vi "Class Map to Plant UML String.vi"(7 "Disabled Set":set{string}(c389), 8 "Usage":bool, 9 "Composition":bool, 10 "Inheritance":bool, 11 "Class Map":T1(c390)) -> (3 "Plant UML String":string)   [LabVIEW 2019]
uses:
  c1262000-356c-4740-a151-1e3da8a0ac02.vi
  72cd38b6-9a28-47ee-a1ef-5582ba5405b3.vi
  38964770-3a7b-4feb-bb65-44f835b9f33f.vi
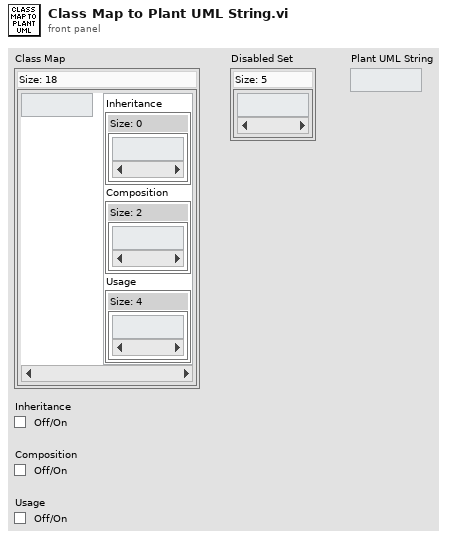
[diagram p1: front panel]
types:
  T1 = map{string, cluster{"Inheritance":set{string}, "Composition":set{string}, "Usage":set{string}}}
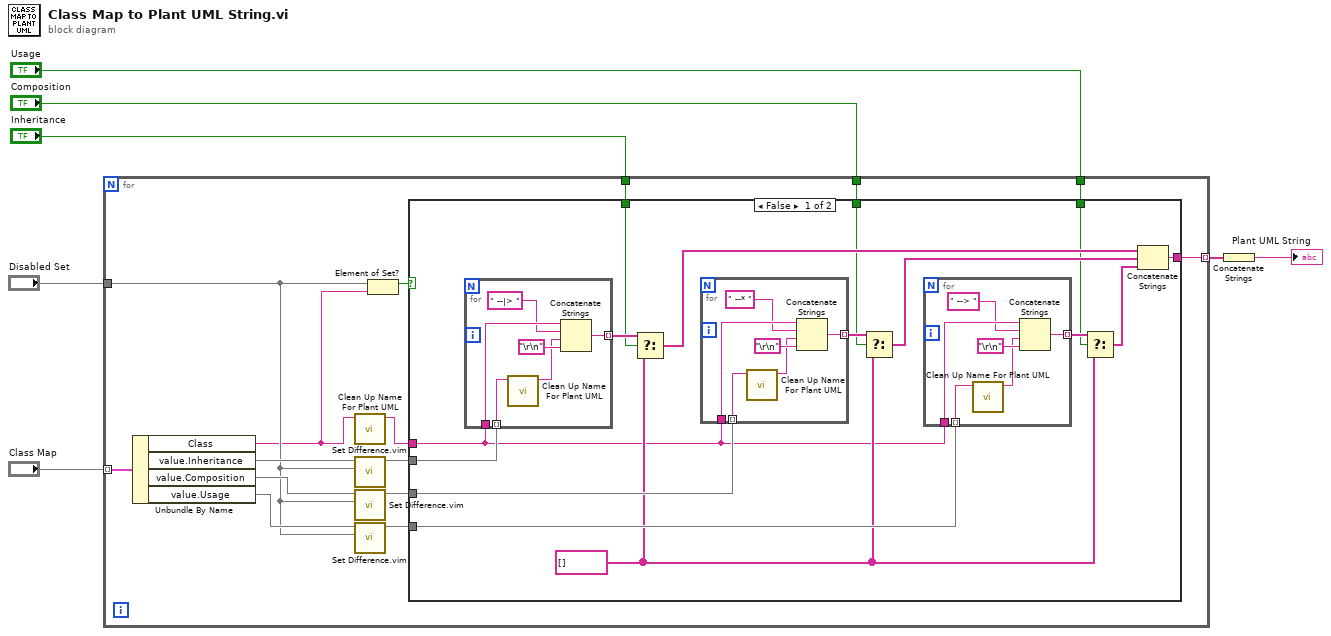
[diagram p0: block diagram]
diagram:
  n1 = for {
    tunnel: "Class Map" -> [w22] mode=indexing
    tunnel: [w21] -> w2 mode=indexing
    tunnel: "Inheritance" -> [w20]
    tunnel: "Composition" -> [w19]
    tunnel: "Usage" -> [w18]
    tunnel: "Disabled Set" -> [w10]
    n2 = Unbundle By Name(w22) -> ("Class"=w9:string, "value.Inheritance"=w16:set{string}, "value.Composition"=w13:set{string}, "value.Usage"=w11:set{string})
    n3 = call "Clean Up Name For Plant UML.vi"("Class Name"=w9) -> ("Plant UML Class Name"=w8:string)  [unwired: 10 in]
    n4 = call "Set Difference.vim"("set 2"=w10, "set 1"=w16) -> ("difference"=w15:set{string})  [unwired: 9 in]
    n5 = call "Set Difference.vim"("set 2"=w10, "set 1"=w13) -> ("difference"=w14:set{string})  [unwired: 9 in]
    n6 = call "Set Difference.vim"("set 2"=w10, "set 1"=w11) -> ("difference"=w12:set{string})  [unwired: 9 in]
    n7 = Element of Set?(10:w9, 11:w10) -> (3:w17:bool)
    n8 = case shown="False" w17 {
      tunnel: w15 -> [w37 _]
      tunnel: w14 -> [w36 _]
      tunnel: w12 -> [w35 _]
      tunnel: [w34 _] -> w21
      tunnel: w20 -> [w26 _]
      tunnel: w19 -> [w25 _]
      tunnel: w18 -> [w24 _]
      tunnel: w8 -> [w23 _]
      frame False {
        w28 = string[] [] ("f")
        n9 = for {
          tunnel: w23 -> [w55]
          tunnel: w37 -> [w51] mode=indexing
          tunnel: [w52] -> w33 mode=indexing
          n10 = call "Clean Up Name For Plant UML.vi"("Class Name"=w51) -> ("Plant UML Class Name"=w50:string)  [unwired: 10 in]
          n11 = Concatenate Strings(w55, " --|> " ("string"), w50, "\r\n") -> (w52:string)
        }
        n12 = Select(t=w33, s=w26, f=w28) -> (s? t:f=w32:string[])
        n13 = for {
          tunnel: w23 -> [w49]
          tunnel: w36 -> [w45] mode=indexing
          tunnel: [w46] -> w31 mode=indexing
          n14 = call "Clean Up Name For Plant UML.vi"("Class Name"=w45) -> ("Plant UML Class Name"=w44:string)  [unwired: 10 in]
          n15 = Concatenate Strings(w49, " --* " ("string"), w44, "\r\n") -> (w46:string)
        }
        n16 = Select(t=w31, s=w25, f=w28) -> (s? t:f=w30:string[])
        n17 = for {
          tunnel: w23 -> [w43]
          tunnel: w35 -> [w39] mode=indexing
          tunnel: [w40] -> w29 mode=indexing
          n18 = call "Clean Up Name For Plant UML.vi"("Class Name"=w39) -> ("Plant UML Class Name"=w38:string)  [unwired: 10 in]
          n19 = Concatenate Strings(w43, " --> " ("string"), w38, "\r\n") -> (w40:string)
        }
        n20 = Select(t=w29, s=w24, f=w28) -> (s? t:f=w27:string[])
        n21 = Concatenate Strings(w32, w30, w27) -> (w34:string)
      }
      frame True {
      }
    }
  }
  n22 = Concatenate Strings(w2) -> (→"Plant UML String":string)
